vi "cast_to_float.vi"(1 "x":i16) -> (0 "y":sgl)   [LabVIEW 2018, in "posit.lvlib"]
uses:
  posit.lvlib
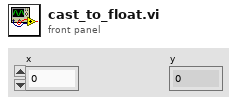
[diagram p1: front panel]
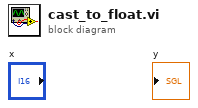
[diagram p0: block diagram]
diagram:
